vi "SSL_CTX_load_verify_locations.vi"(8 "error in (no error)":errorcluster, 10 "Path to CA bundle":path=path "C:/Program Files (x86)/National Instruments/RT Images/nissl/18.0.0/ca-bundle.crt", 11 "SSL-Context in":refnum<class "SSL-Context.lvclass">) -> (0 "error out":errorcluster, 3 "SSL-Context out":refnum<class "SSL-Context.lvclass">)   [LabVIEW 2013, in "SSL_Lib.lvlib" / "SSL-Context.lvclass"]
uses:
  SSL-Context.lvclass
  SSL-Lib/SSL-Lib.lvclass
panel:
  out "return type":i32
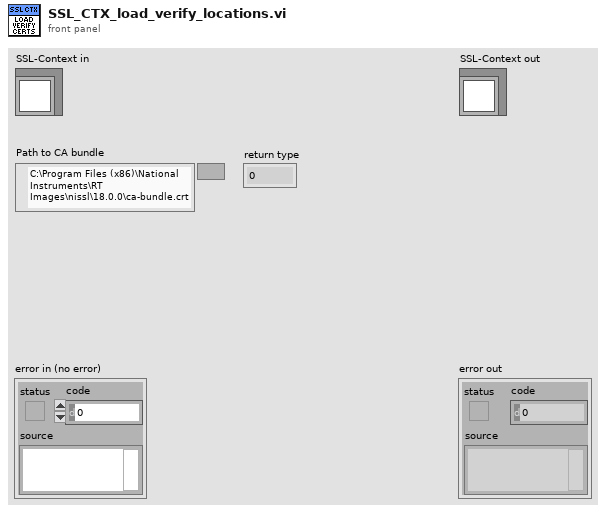
[diagram p1: front panel]
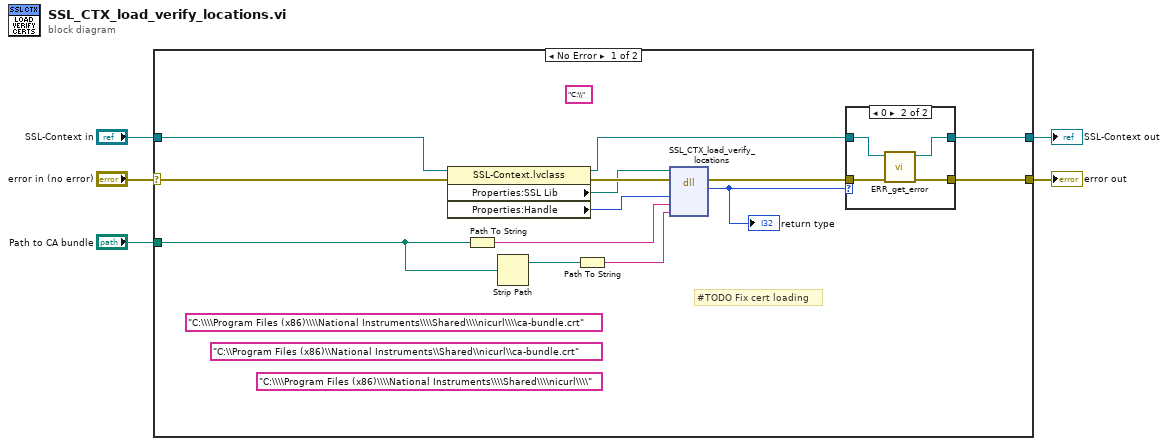
[diagram p0: block diagram]
diagram:
  n1 = case shown="No Error" "error in (no error)" {
    selector: "error in (no error)" -> [w19 w27]
    tunnel: [w11 w27] -> w4
    tunnel: [w12 w26] -> w2
    tunnel: "SSL-Context in" -> [w17 w26]
    tunnel: "Path to CA bundle" -> [w9 _]
    frame No Error {
      (unwired) "C:\\" ("CAFile")
      (unwired) "C:\\\\Program Files (x86)\\\\National Instruments\\\\Shared\\\\nicurl\\\\" ("CAFile")
      (unwired) "C:\\Program Files (x86)\\National Instruments\\Shared\\nicurl\\ca-bundle.crt" ("CAFile")
      (unwired) "C:\\\\Program Files (x86)\\\\National Instruments\\\\Shared\\\\nicurl\\\\ca-bundle.crt" ("CAFile")
      # "#TODO Fix cert loading"
      n2 = property class="SSL-Context.lvclass"(reference=w17, error in=w19) -> (reference out=w13:refnum<class "SSL-Context.lvclass">, error out=w18:errorcluster, "Properties:SSL Lib"=w16:path, "Properties:Handle"=w15:u64)
      n3 = Path To String(path=w9) -> (string=w6:string)
      n4 = Strip Path(path=w9) -> (stripped path=w8:path)  [unwired: 1 out]
      n5 = Path To String(path=w8) -> (string=w7:string)
      n6 = dll-call lib="C:/Program Files (x86)/National Instruments/Shared/nissl/NIssleay32.dll" fn="SSL_CTX_load_verify_locations"(path in=w16, error in=w18, "SSL_CTX"=w15, "CAFile"=w6, "CApath"=w7) -> (error out=w14:errorcluster, "return type"=w10:i32)  [unwired: 4 in, 1 out]
      "return type" <- w10
      n7 = case shown="0" w10 {
        tunnel: w14 -> [w21 w25]
        tunnel: w13 -> [w20 w24]
        tunnel: [w20 w23] -> w12
        tunnel: [w21 w22] -> w11
        frame Default {
        }
        frame 0 {
          n8 = call "ERR_get_error.vi"("error in (no error)"=w25, "SSL-Lib in"=w24) -> ("error out"=w22:errorcluster, "SSL-Lib out"=w23:refnum<class "SSL-Context.lvclass">)  [unwired: 8 in]
        }
      }
    }
    frame Error {
    }
  }
  "error out" <- w4
  "SSL-Context out" <- w2
